vi "LV SciSDK INIT FFT.vi"(0 "FFT Name":string, 1 "Acq mode":string(combo)="blocking", 5 "Decimator":u32, 7 "Timeout":i32=5000, 9 "Board Handle In":T1, 11 "error in (no error)":errorcluster) -> (8 "FFT Handle Out":cluster{"FFT Path":string, "FFT Name":string}, 10 "Board Handle Out":T1, 15 "error out":errorcluster)   [LabVIEW 2021, in "SciSDK_Labview.lvlib"]
uses:
  SciSDK_Labview.lvlib
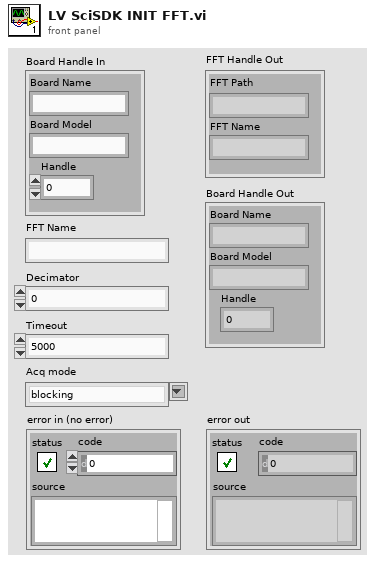
[diagram p1: front panel]
types:
  T1 = cluster{"Board Name":string, "Board Model":string, "Handle":u64}
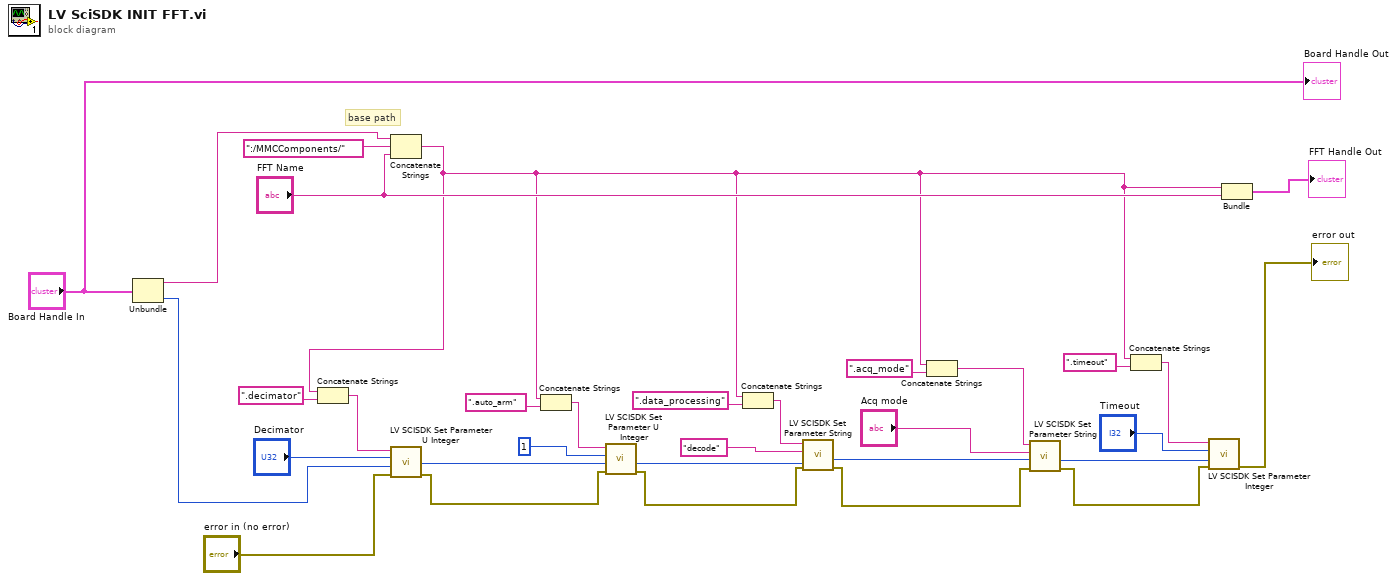
[diagram p0: block diagram]
diagram:
  # "base path"
  n1 = Unbundle("Board Handle In") -> ("Board Name"=w31:string, "Handle"=w22:u64)  [unwired: 1 out]
  n2 = Concatenate Strings(w31, ":/MMCComponents/" ("string"), "FFT Name") -> (w2:string)
  n3 = Concatenate Strings(w2, ".decimator" ("string")) -> (w21:string)
  n4 = call "LV SCISDK Set Parameter U Integer.vi"("error in (no error)"="error in (no error)", "handle"=w22, "value"="Decimator", "Path"=w21) -> ("error out"=w17:errorcluster, "handle out"=w18:u64)  [unwired: 5 in, 1 out]
  n5 = Concatenate Strings(w2, ".auto_arm" ("string")) -> (w19:string)
  n6 = call "LV SCISDK Set Parameter U Integer.vi"("error in (no error)"=w17, "handle"=w18, "value"=u32 1, "Path"=w19) -> ("error out"=w15:errorcluster, "handle out"=w16:u64)  [unwired: 5 in, 1 out]
  n7 = Concatenate Strings(w2, ".data_processing" ("string")) -> (w13:string)
  n8 = call "LV SCISDK Set Parameter String.vi"("error in (no error)"=w15, "handle"=w16, "value"="decode", "Path"=w13) -> ("error out"=w12:errorcluster, "handle out"=w11:u64)  [unwired: 5 in, 1 out]
  n9 = Concatenate Strings(w2, ".acq_mode" ("string")) -> (w9:string)
  n10 = call "LV SCISDK Set Parameter String.vi"("error in (no error)"=w12, "handle"=w11, "value"="Acq mode", "Path"=w9) -> ("error out"=w4:errorcluster, "handle out"=w5:u64)  [unwired: 5 in, 1 out]
  n11 = Concatenate Strings(w2, ".timeout" ("string")) -> (w7:string)
  n12 = call "LV SCISDK Set Parameter Integer.vi"("error in (no error)"=w4, "handle"=w5, "value"="Timeout", "Path"=w7) -> ("error out"=→"error out":errorcluster)  [unwired: 5 in, 2 out]
  n13 = Bundle(w2, "FFT Name"="FFT Name") -> (→"FFT Handle Out":cluster{string, "FFT Name":string})  [unwired: 1 in]
  "Board Handle Out" <- "Board Handle In"
